vi "clearpath_parse_encoder.vi"(5 "ClearpathComm":T1) -> (0 "Left Distance (m)":dbl, 1 "Right Distance (m)":dbl, 2 "Left Speed (m/s)":dbl, 3 "Right Speed (m/s)":dbl, 4 "Data Valid?":bool=TRUE)   [LabVIEW 2012, in "clearpath_interface.lvlib"]
doc: "Parses encoder data. Encoder data has been converted to real-world units. (Message type 0x8800)"
uses:
  clearpath_interface.lvlib
  cwrap_crio.dll
panel:
  # "Encoder Data"
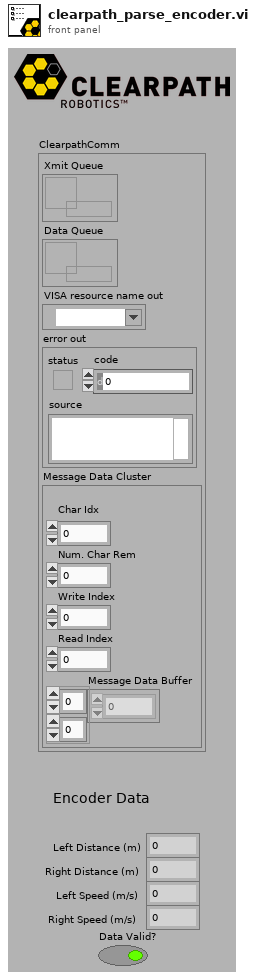
[diagram p1: front panel]
types:
  T1 = cluster{"Xmit Queue":refnum<queue>, "Data Queue":refnum<queue>, "VISA resource name out":refnum<visa-resource-name>, "error out":errorcluster, "Message Data Cluster":cluster{"\nChar Idx":u8, "Num. Char Rem":u8, "Write Index":u8, "Read Index":u8, "Message Data Buffer":u8[][]}}
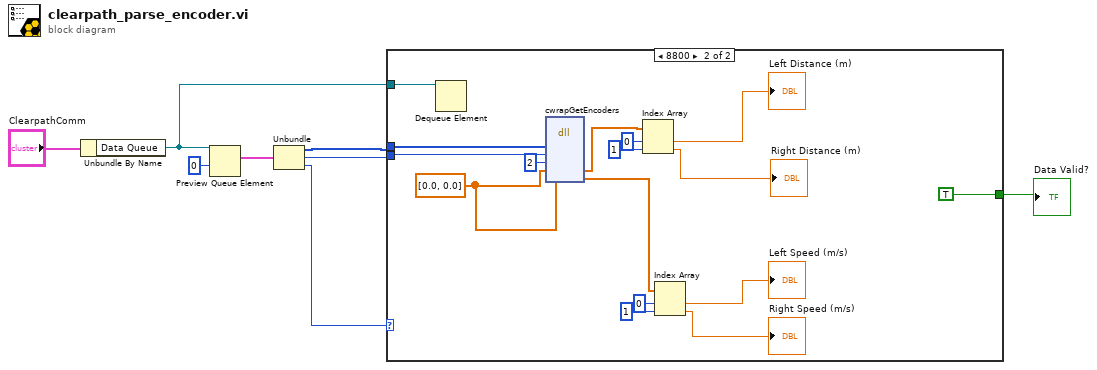
[diagram p0: block diagram]
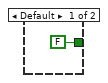
[diagram p2: hidden frame]
diagram:
  n1 = Unbundle By Name("ClearpathComm") -> ("Data Queue"=w1:refnum<queue>)
  n2 = Preview Queue Element(queue=w1, timeout in ms (-1)=0) -> (element=w6:cluster{u8[], "Length":i32, "Type":i32})  [unwired: 1 in, 3 out]
  n3 = Unbundle(w6) -> (w3:u8[], "Length"=w4:i32, "Type"=w5:i32)
  n4 = case shown="8800" w5 {
    tunnel: w4 -> [_ w12]
    tunnel: w3 -> [_ w13]
    tunnel: [FALSE TRUE] -> w2
    tunnel: w1 -> [_ w10]
    frame Default {
    }
    frame 34816 {
      w24 = dbl[] [0.0, 0.0] ("Array")
      n5 = Dequeue Element(queue=w10) -> ()  [unwired: 2 in, 4 out]
      n6 = dll-call lib="C:/Users/cartersm/Documents/GitHub/IGVC-2013/Code/Project 1.0/Motors/Husky/cwrap_cRIO.*" fn="cwrapGetEncoders"("packet"=w13, "len"=w12, "enc_count"=i8 2, "travel"=w24, "speed"=w24) -> ("travel"=w21:dbl[], "speed"=w18:dbl[])  [unwired: 7 in, 2 out]
      n7 = Index Array(array=w21, index #1=0 ("index"), index #2=1 ("index")) -> (element #1=→"Left Distance (m)":dbl, element #2=→"Right Distance (m)":dbl)
      n8 = Index Array(array=w18, index #1=0 ("index"), index #2=1 ("index")) -> (element #1=→"Left Speed (m/s)":dbl, element #2=→"Right Speed (m/s)":dbl)
    }
  }
  "Data Valid?" <- w2
